vi "Flatten.vi"(6 "FIFO Timestamps":T2, 8 "error in (no error)":errorcluster, 10 "Data In":T1[](array[typedef]), 11 "CIF_NIChn_FIFO_DAQ in":refnum<class "CIF_NIChn_FIFO_DAQ.lvclass">) -> (0 "error out":errorcluster, 2 "Data Out":T1[](array[typedef]), 3 "CIF_NIChn_FIFO_DAQ out":refnum<class "CIF_NIChn_FIFO_DAQ.lvclass">)   [LabVIEW 2021, in "CIF_NIChn_FIFO_DAQ.lvclass"]
uses:
  CIF_NIChn_FIFO_DAQ.lvclass
  D:/dev/Packages/Channel_Manager/src/CIFChannels/CIFChannels.lvclass
  D:/dev/Packages/Channel_Manager/src/CIF_NIChn/FIFO_U8/CIF_NIChn_Fifo_U8.lvclass
  ChannelCommon/typedef/TimeStamps.ctl
  ChannelCommon/typedef/Datatype Waveform.ctl
  CIFChannels/CIFChannels.lvclass/CIFChannels.ctl
  CIF_NIChn_FIFO_DAQ.lvclass/CIF_NIChn_FIFO_DAQ.ctl
  FIFO_U8/CIF_NIChn_Fifo_U8.lvclass/CIF_NIChn_Fifo_U8.ctl
  <vilib>/CIF Foundation/CIF Utilities/Statistics/I64/Stats_I64_CIF_U.lvclass/Stats_I64_CIF_U.ctl
  FIFO_U8/Accessors/Read Payload.vi
  FIFO_U8/Accessors/Write Payload.vi
  587a020d-d764-4ff7-9451-6b801beca2fa.vi
  b511efe2-f594-4971-95dc-73ac55586360.vi
  CIFChannels/Accessors/Read FIFO Retry on Timeout.vi
  <vilib>/CIF Foundation/CIF Utilities/DataTypes/Flatten U64.vi
  CIFChannels/Utilities/Create Flattened FIFO Header.vi
  <vilib>/CIF Foundation/CIF Utilities/Statistics/I64/X1 minus X0.vi
  <vilib>/CIF Foundation/CIF Utilities/Time/System Time/Get System Time.vi
  ChannelCommon/Utilities/Flatten Header.vi
  CIFChannels/Utilities/Update FIFO Header.vi
  <vilib>/CIF Foundation/CIF Utilities/Statistics/I64/X1 minus X0.vi/dfabcf33-0dbc-4041-80a5-3dc0c86d2989.vi
  <vilib>/CIF Foundation/CIF Utilities/Time/System Time/LabVIEW Time to TAI Time.vi
  <vilib>/CIF Foundation/CIF Utilities/DataTypes/Flatten I64.vi
  <vilib>/CIF Foundation/CIF Utilities/Statistics/I64/X1 minus X0.vi/dfabcf33-0dbc-4041-80a5-3dc0c86d2989.vi/9eb60a9a-770f-4d2d-8b3f-8465c267ecc9.vi
  CIFChannels/CIFChannels.lvclass
  D:/dev/Packages/Channel_Manager/src/CIF_NIChn/NIChn/CIF_NIChn.lvclass
  D:/dev/Packages/Channel_Manager/src/CIF_NIChn/FIFO_DAQ  not DVR/CIF_NIChn_FIFO_DAQ.lvclass
  ChannelCommon/ChannelCommon.lvlib
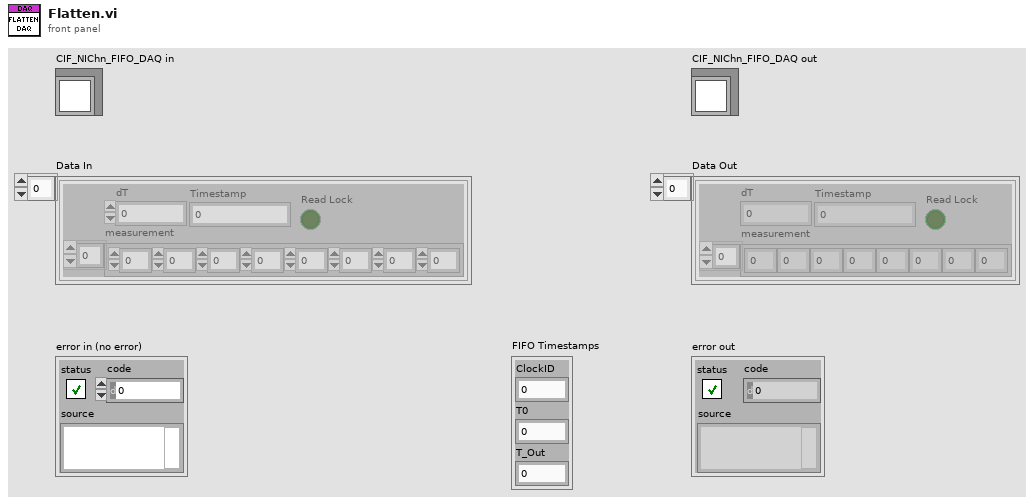
[diagram p1: front panel]
types:
  T1 = typedef "ChannelCommon.lvlib/Datatype Waveform.ctl" = cluster{"measurement":dbl[], "dT":dbl, "Timestamp":i64, "Read Lock":bool}
  T2 = typedef "ChannelCommon.lvlib/TimeStamps.ctl" = cluster{"ClockID":u8, "T0":i64, "T_Out":i64}
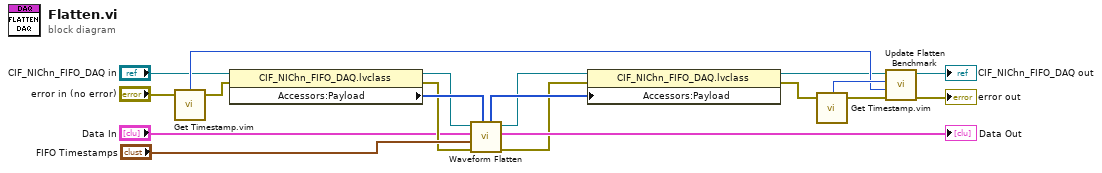
[diagram p0: block diagram]
diagram:
  n1 = call "Get Timestamp.vim"("Anything in"="error in (no error)") -> ("Time (ns)"=w13:i64, "Anything out"=w14:errorcluster)  [unwired: 2 in]
  n2 = property class="CIF_NIChn_FIFO_DAQ.lvclass"(reference="CIF_NIChn_FIFO_DAQ in", error in=w14) -> (reference out=w8:refnum<class "CIF_NIChn_FIFO_DAQ.lvclass">, error out=w9:errorcluster, "Accessors:Payload"=w11:u8[])
  n3 = call "Waveform Flatten.vi"("payload in"=w11, "error in (no error)"=w9, "FIFO Timestamps"="FIFO Timestamps", "Data in"="Data In", "CIFChannels in"=w8) -> ("error out"=w3:errorcluster, "Data out"=→"Data Out":T1[], "CIFChannels out"=w1:refnum<class "CIF_NIChn_FIFO_DAQ.lvclass">, "payload out"=w7:u8[])  [unwired: 2 in, 1 out]
  n4 = property class="CIF_NIChn_FIFO_DAQ.lvclass"(reference=w1, error in=w3, "Accessors:Payload"=w7) -> (reference out=w4:refnum<class "CIF_NIChn_FIFO_DAQ.lvclass">, error out=w2:errorcluster)
  n5 = call "Get Timestamp.vim"("Anything in"=w2) -> ("Time (ns)"=w16:i64, "Anything out"=w17:errorcluster)  [unwired: 2 in]
  n6 = call "Update Flatten Benchmark.vi"("error in (no error)"=w17, "X0"=w13, "X1"=w16, "CIFChannels in"=w4) -> ("error out"=→"error out":errorcluster, "CIFChannels out"=→"CIF_NIChn_FIFO_DAQ out":refnum<class "CIF_NIChn_FIFO_DAQ.lvclass">)  [unwired: 6 in]
